vi "RichToFlatnixnet_grpc_WriteSignalSinglePointResponse.vi"(5 "OutputClusterType":T1, 11 "InputCluster":T2) -> (3 "OutputCluster":T1)   [LabVIEW 2025, in "grpc-xnet_client.lvlib"]
uses:
  nixnet_grpc_WriteSignalSinglePointResponse.ctl
  nixnet_grpc_WriteSignalSinglePointResponse_Flat.ctl
  grpc-xnet_client.lvlib
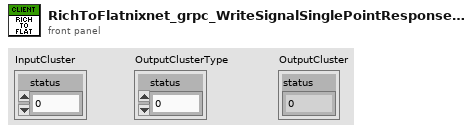
[diagram p1: front panel]
types:
  T1 = typedef "grpc-xnet_client.lvlib/nixnet_grpc_WriteSignalSinglePointResponse_Flat.ctl" = cluster{"status":i32}
  T2 = typedef "grpc-xnet_client.lvlib/nixnet_grpc_WriteSignalSinglePointResponse.ctl" = cluster{"status":i32}
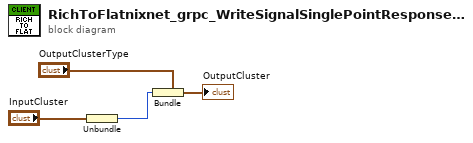
[diagram p0: block diagram]
diagram:
  n1 = Unbundle "Unbundle"("InputCluster") -> ("status"=w1:i32)
  n2 = Bundle "Bundle"(cluster="OutputClusterType", "status"=w1) -> (→"OutputCluster":T1)
